vi "Navigate - copy.vi"(1 "Pathfinding Settings":T1={"Movement Settings"={"Arrival Tolerance (m)"=0.01, "Closeness Threshold (m)"=0.5, "Pit Obstacle Radius (m)"=0.5, "Pit Locations"=[]}, "Dead Zone"=0.75, "Max Moves"=3.0, "Move Segment Length (m)"=0.02, "Path Cost Weights"={"Length Weight"=1.0, "Angle Weight"=0.0, "Angle Error Weight"=1000.0, "Angle Error Threshold"=0.314, "Per Move Penalty"=0.05, "Closeness Weight"=100.0, "Too Short Penalty"=100.0, "Too Short Threshold"=1.5}, "Desperation - Reduction Per Attempt (Ratio)"=0.9, "Desperation - Max Attempts"=1, "Log All Move Points"=FALSE, "Intermediate Position Grids"=[{"x1"=0.0, "x2"=1.75, "resolution"=0.15}, {"x1"=1.75, "x2"=7.38, "resolution"=0.4}]}, 2 "Move Type":T5(ring)) -> ()   [LabVIEW 2015, in "Navigation2017.lvlib"]
uses:
  Navigation2017.lvlib
  Vector.ctl
  PathOfMoves.ctl
  Move.ctl
  Navigation2017-util.lvlib
  PathfindingSettings.ctl
  MovementSettings.ctl
  PathCostWeights.ctl
  IntermediatePositionGrids.ctl
panel:
  out "Pathfinding Loop Count":i32
  in  "Reached Next Path Point Threshold Distance (m)":dbl(knob)=0.2054620332336267 scale=0.0..1.0
  in  "Robot Speed":dbl(slide)=1.0 scale=0.0..1.0
  in  "Dead Reckoning Move Distance (m)":dbl(knob)=1.1303212530968743 scale=0.5..4.0
  in  "Turning Radius (m)":dbl(knob)=0.75 scale=0.75..4.0
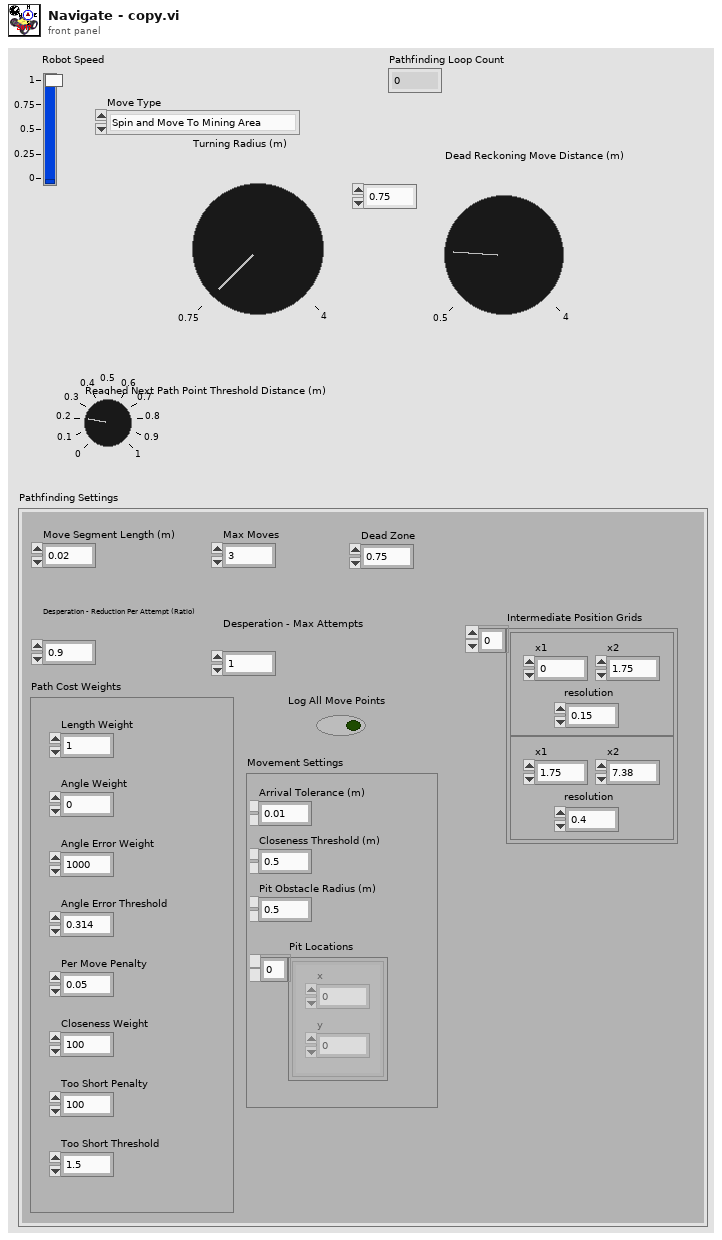
[diagram p1: front panel]
types:
  T1 = typedef "Navigation2017.lvlib/PathfindingSettings.ctl" = cluster{"Movement Settings":T2, "Dead Zone":dbl, "Max Moves":dbl, "Move Segment Length (m)":dbl, "Path Cost Weights":T3, "Desperation - Reduction Per Attempt (Ratio)":dbl, "Desperation - Max Attempts":i16, "Log All Move Points":bool, "Intermediate Position Grids":T4}
  T2 = typedef "Navigation2017.lvlib/MovementSettings.ctl" = cluster{"Arrival Tolerance (m)":dbl, "Closeness Threshold (m)":dbl, "Pit Obstacle Radius (m)":dbl, "Pit Locations":cluster{"x":dbl, "y":dbl}[]}
  T3 = typedef "Navigation2017.lvlib/PathCostWeights.ctl" = cluster{"Length Weight":dbl, "Angle Weight":dbl, "Angle Error Weight":dbl, "Angle Error Threshold":dbl, "Per Move Penalty":dbl, "Closeness Weight":dbl, "Too Short Penalty":dbl, "Too Short Threshold":dbl}
  T4 = typedef "Navigation2017.lvlib/IntermediatePositionGrids.ctl" = cluster{"x1":dbl, "x2":dbl, "resolution":dbl}[]
  T5 = enum16{"Spin and Move To Mining Area", "Move To Collector Trough", "Move To Mining Area"}
  T6 = typedef "Navigation2017.lvlib/Vector.ctl" = cluster{"x":dbl, "y":dbl, "angle":dbl}
  T7 = typedef "LocalizationStatus.ctl" = cluster{"x":dbl, "y":dbl, "angle":dbl, "valid":bool, "lastUpdatedTime":dbl}
  T8 = typedef "Navigation2017.lvlib/PathOfMoves.ctl" = cluster{"Dest Angle Error":dbl, "Dest Angle Considered":bool, "Moves":T9[]}
  T9 = typedef "Navigation2017.lvlib/Move.ctl" = cluster{"Did Reach Dest":bool, "Did Collide":bool, "Sum of Angle Changes (rad)":dbl, "Move Length (m)":dbl, "Closeness Sum":dbl, "Positions Along Move":T6[], "Moved Fwd":bool}
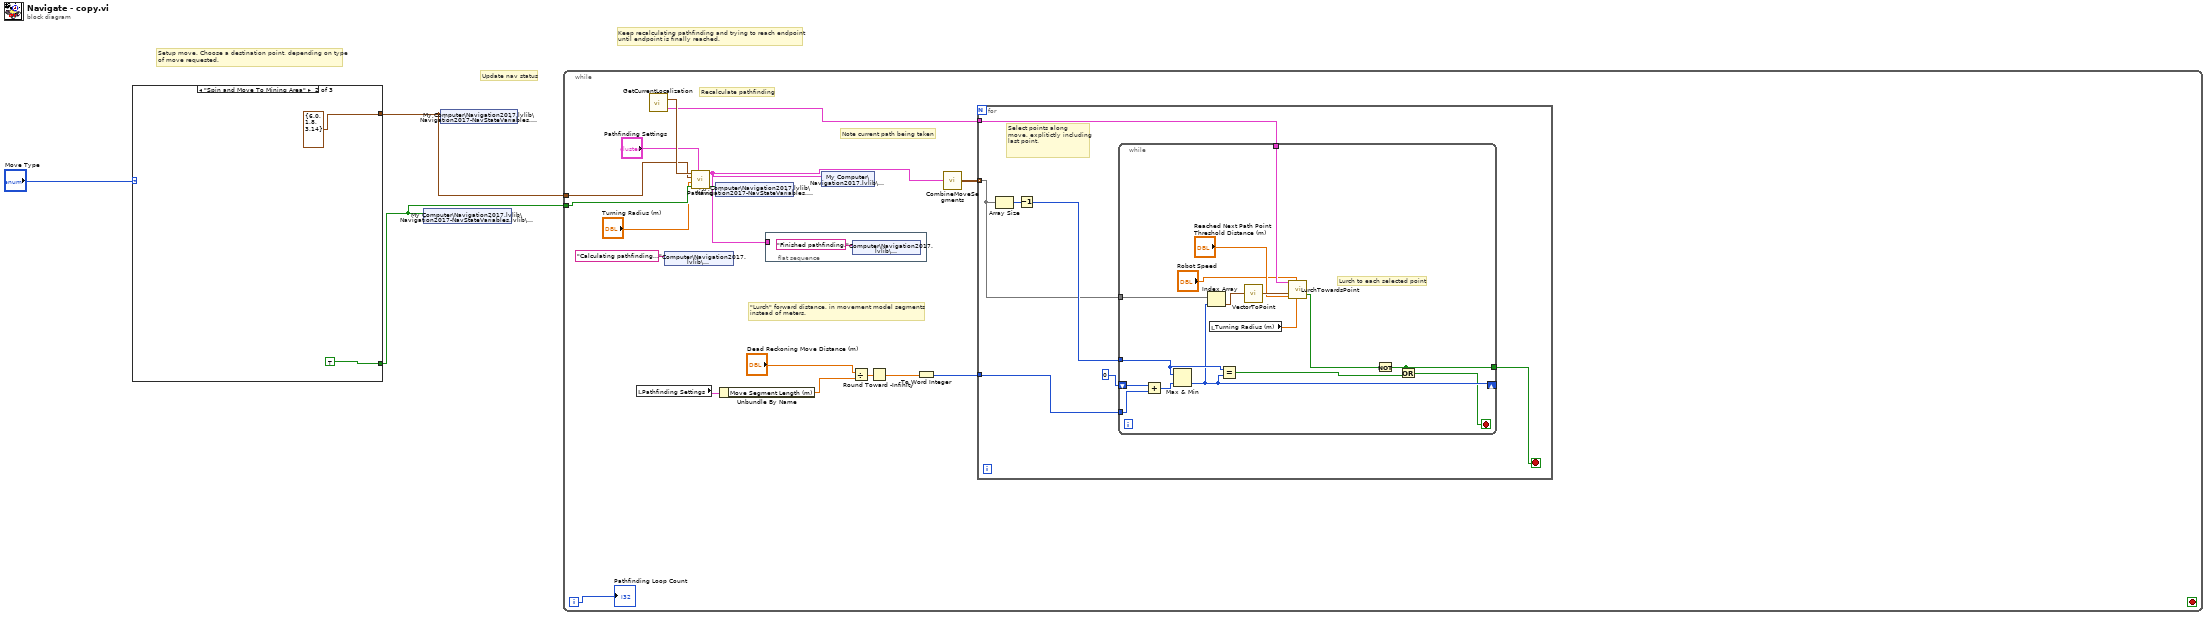
[diagram p0: block diagram]
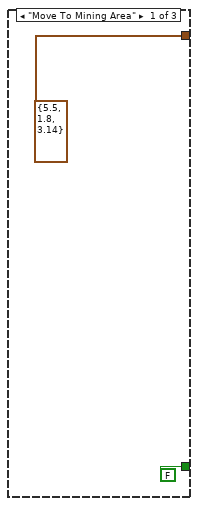
[diagram p2: hidden frame]
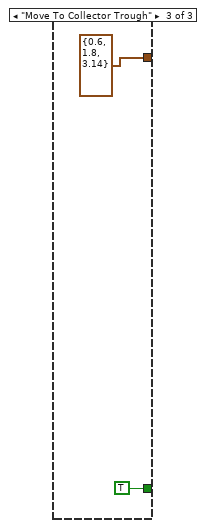
[diagram p3: hidden frame]
diagram:
  # "Keep recalculating pathfinding and trying to reach endpoint\nuntil endpoint is finally reached."
  # "Update nav status"
  # "Setup move. Choose a destination point, depending on type\nof move requested."
  n1 = case shown="\"Spin and Move To Mining Area\"" "Move Type" {
    tunnel: [T6 {"x"=5.5, "y"=1.8, "angle"=3.14} ("Vector") T6 {"x"=6.0, "y"=1.8, "angle"=3.14} ("Vector") T6 {"x"=0.6, "y"=1.8, "angle"=3.14} ("Vector")] -> w2
    tunnel: [FALSE TRUE TRUE] -> w1
    frame "Move To Mining Area" {
    }
    frame "Spin and Move To Mining Area" {
    }
    frame "Move To Collector Trough" {
    }
  }
  n2 = shared-variable "My Computer\\Navigation2017.lvlib\\Navigation2017-NavStateVariables.lvlib\\SpecifyingEndAngle"(w1) -> ()  [unwired: 1 in, 1 out]
  n3 = shared-variable "My Computer\\Navigation2017.lvlib\\Navigation2017-NavStateVariables.lvlib\\DestinationPoint"(w2) -> ()  [unwired: 1 in, 1 out]
  n4 = while {
    tunnel: w2 -> [w24]
    tunnel: w1 -> [w23]
    i -> [w26]
    stop <- _ stop-if-true
    # "\"Lurch\" forward distance, in movement model segments\ninstead of meters."
    # "Note current path being taken"
    # "Recalculate pathfinding"
    n5 = local read "Pathfinding Settings"() -> (w15:T1)
    n6 = call "GetCurrentLocalization.vi"() -> ("Current Localization Status"=w10:T7, "Current Localization Vector"=w25:T6)
    n7 = shared-variable "My Computer\\Navigation2017.lvlib\\Navigation2017-NavStateVariables.lvlib\\CurrNavStage"("Calculating pathfinding..." ("CurrNavStage")) -> ()  [unwired: 1 in, 1 out]
    n8 = call "Pathfind.vi"("Pathfinding Settings"="Pathfinding Settings", "Specified End Angle"=w23, "Turn Radius (m)"="Turning Radius (m)", "Destination"=w24, "Start Vector"=w25) -> ("Desperation Used"=w20:bool, "Best Path"=w14:T8)  [unwired: 3 out]
    n9 = shared-variable "My Computer\\Navigation2017.lvlib\\Navigation2017-NavStateVariables.lvlib\\UsedDesperation"(w20) -> ()  [unwired: 1 in, 1 out]
    n10 = Unbundle By Name(w15) -> ("Move Segment Length (m)"=w16:dbl)
    n11 = flat-sequence {
      tunnel: w14 -> [_]
      frame #0 {
        n12 = shared-variable "My Computer\\Navigation2017.lvlib\\Navigation2017-NavStateVariables.lvlib\\CurrNavStage"("Finished pathfinding." ("CurrNavStage")) -> ()  [unwired: 1 in, 1 out]
      }
    }
    n13 = shared-variable "My Computer\\Navigation2017.lvlib\\Navigation2017-NavStateVariables.lvlib\\CurrPath"(w14) -> ()  [unwired: 1 in, 1 out]
    n14 = Divide(x="Dead Reckoning Move Distance (m)", y=w16) -> (x/y=w18:dbl)
    n15 = Round Toward -Infinity(1:w18) -> (0:w11:dbl)
    n16 = To Word Integer(number=w11) -> (16bit integer=w12:i16)
    n17 = call "CombineMoveSegments.vi"("Path"=w14) -> ("Combined Moves and Segments"=w13:T6[][])
    n18 = for {
      tunnel: w13 -> [w29] mode=indexing
      tunnel: w12 -> [w33]
      tunnel: w10 -> [w28]
      stop <- w27 stop-if-true
      # "Select points along\nmove, explitictly including last point."
      n19 = Array Size(array=w29) -> (size(s)=w31:i32)
      n20 = Decrement(x=w31) -> (x-1=w30:i32)
      n21 = while {
        shift-right: [w44] -> _
        shift-left: i16 0 -> [w48]
        tunnel: w33 -> [w49]
        tunnel: w30 -> [w46]
        tunnel: w29 -> [w43]
        tunnel: w28 -> [w41]
        tunnel: [w34] -> w27
        stop <- w35 stop-if-true
        # "Lurch to each selected point"
        n22 = Add(x=w48, y=w49) -> (x+y=w47:i32)
        n23 = Max & Min(x=w46, y=w47) -> (min(x,y)=w44:i32)  [unwired: 1 out]
        n24 = Index Array(array=w43, index=w44) -> (element=w42:T6)
        n25 = local read "Turning Radius (m)"() -> (w38:dbl)
        n26 = Equal?(x=w46, y=w44) -> (x = y?=w36:bool)
        n27 = call "VectorToPoint.vi"("Vector"=w42) -> ("Point"=w45:cluster{"x":dbl, "y":dbl})
        n28 = call "LurchTowardsPoint.vi"("Turning Radius (m)"=w38, "Robot Speed"="Robot Speed", "Reached Next Path Point Threshold Distance (m)"="Reached Next Path Point Threshold Distance (m)", "Dest. Point"=w45, "Curr Localization Status"=w41) -> ("Within Tolerance of Dest"=w37:bool)  [unwired: 1 in, 1 out]
        n29 = Not(x=w37) -> (.not. x?=w34:bool)
        n30 = Or(x=w34, y=w36) -> (x .or. y?=w35:bool)
      }
    }
    "Pathfinding Loop Count" <- w26
  }
